vi "RW Test.vi"() -> (0 "error out":errorcluster, 2 "Pass":bool)   [LabVIEW 2021]
uses:
  Zenoh.lvclass/Zenoh.ctl
  Wrappers/Put Raw Wrapper.vi
  Core/Write Double.vi/58400e5e-2cc1-4aca-8f0f-3a78c0a2476e.vi
  Wrappers/Poll Raw Wrapper.vi
  Core/Read Double.vi/4c4e9aed-29a9-49a4-ae79-bb096e87db4b.vi
  SubVIs/Get Zenoh Path.vi
  Core/Write Double.vi/58400e5e-2cc1-4aca-8f0f-3a78c0a2476e.vi/c28b0ead-42ad-4072-80a2-aca7f2bd7ce3.vi
  Core/Write Double.vi/58400e5e-2cc1-4aca-8f0f-3a78c0a2476e.vi/d83f0d1e-b5f2-409c-a855-55c666a7c55e.vi
  Core/Write Double.vi/58400e5e-2cc1-4aca-8f0f-3a78c0a2476e.vi/e02991d1-a06a-4e5e-a573-6dce97b92612.vi
  Core/Read Double.vi/4c4e9aed-29a9-49a4-ae79-bb096e87db4b.vi/c28b0ead-42ad-4072-80a2-aca7f2bd7ce3.vi
  Core/Read Double.vi/4c4e9aed-29a9-49a4-ae79-bb096e87db4b.vi/48104490-ec73-4168-8754-ff252ec03617.vi
  <vilib>/CIF Foundation/CIF Utilities/DataTypes/SubVIs/DataTypes Error.vi
  Core/Read Double.vi/4c4e9aed-29a9-49a4-ae79-bb096e87db4b.vi/543c0f61-77eb-4f29-b175-1688c1700ba4.vi
  <vilib>/CIF Foundation/CIF Utilities/DataTypes/SubVIs/DataTypes Error Core.vi
  Zenoh.lvclass
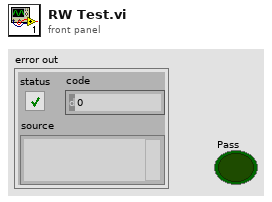
[diagram p1: front panel]
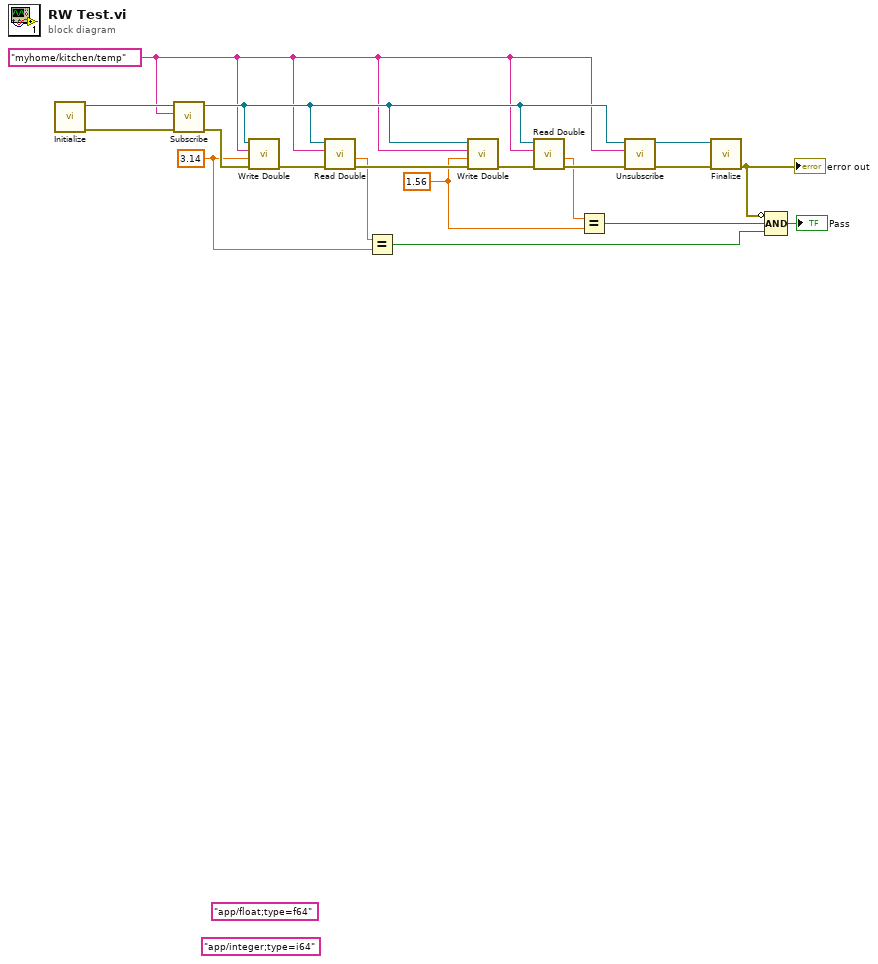
[diagram p0: block diagram]
diagram:
  w8 = 1.56 ("Numeric")
  w10 = 3.14 ("Numeric")
  w2 = "myhome/kitchen/temp" ("key")
  (unwired) "app/integer;type=i64" ("value")
  (unwired) "app/float;type=f64" ("value")
  n1 = call "Initialize.vi"() -> ("error out"=w19:errorcluster, "Zenoh out"=w18:refnum<class "Zenoh.lvclass">)  [unwired: 10 in]
  n2 = call "Subscribe.vi"("error in (no error)"=w19, "Key"=w2, "Zenoh in"=w18) -> ("error out"=w17:errorcluster, "Zenoh out"=w12:refnum<class "Zenoh.lvclass">)  [unwired: 7 in]
  n3 = call "Write Double.vi"("error in (no error)"=w17, "Numeric"=w10, "Key"=w2, "Zenoh in"=w12) -> ("error out"=w16:errorcluster)  [unwired: 7 in]
  n4 = call "Read Double.vi"("error in (no error)"=w16, "Key"=w2, "Zenoh in"=w12) -> ("error out"=w15:errorcluster, "Numeric Out"=w11:dbl)  [unwired: 6 in, 1 out]
  n5 = Equal?(x=w11, y=w10) -> (x = y?=w7:bool)
  n6 = call "Write Double.vi"("error in (no error)"=w15, "Numeric"=w8, "Key"=w2, "Zenoh in"=w12) -> ("error out"=w14:errorcluster)  [unwired: 7 in]
  n7 = call "Read Double.vi"("error in (no error)"=w14, "Key"=w2, "Zenoh in"=w12) -> ("error out"=w13:errorcluster, "Numeric Out"=w9:dbl)  [unwired: 6 in, 1 out]
  n8 = Equal?(x=w9, y=w8) -> (x = y?=w6:bool)
  n9 = call "Unsubscribe.vi"("error in (no error)"=w13, "Key"=w2, "Zenoh in"=w12) -> ("error out"=w1:errorcluster, "Zenoh out"=w3:refnum<class "Zenoh.lvclass">)  [unwired: 7 in]
  n10 = call "Finalize.vi"("error in (no error)"=w1, "Zenoh in"=w3) -> ("error out"=w5:errorcluster)  [unwired: 8 in, 1 out]
  "error out" <- w5
  n11 = Compound Arithmetic op=AND(invert w5, w6, w7) -> (→"Pass":bool)
